vi "Application Stop.vi"() -> ()   [LabVIEW 2020]
panel:
  in  "Application Global Stop":bool
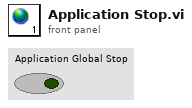
[diagram p1: front panel]
diagram:
